vi "Read Synch.vi"(8 "error in (no error)":errorcluster, 11 "AnalogInput in":refnum<class "AnalogInput.lvclass">) -> (0 "error out":errorcluster, 2 "Timing":T1={"Source"="", "Sample Rate (10k)"=10000.0, "sample mode"=10178, "samples per channel"=1000} {"sample mode" items=["Finite Samples"=10178, "Continuous Samples"=10123, "Hardware Timed Single Point"=12522]}, 3 "AnalogInput out":refnum<class "AnalogInput.lvclass">)   [LabVIEW 2019, in "AnalogInput.lvlib" / "AnalogInput.lvclass"]
uses:
  Library/AnalogInput.lvclass
  Custom Controls/Synch Settings.ctl
  Library/AnalogInput.lvclass/AnalogInput.ctl
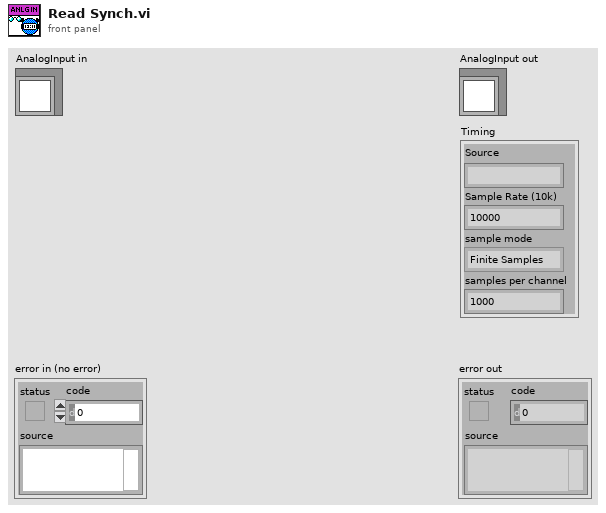
[diagram p1: front panel]
types:
  T1 = typedef "AnalogInput.lvlib/AnalogInput.lvclass/Synch Settings.ctl" = cluster{"Source":string, "Sample Rate (10k)":dbl, "sample mode":i32, "samples per channel":i32}
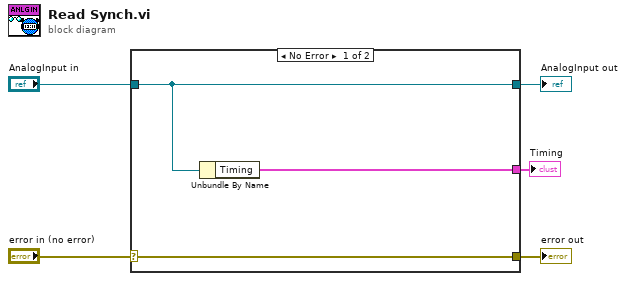
[diagram p0: block diagram]
diagram:
  n1 = case shown="No Error" "error in (no error)" {
    selector: "error in (no error)" -> [w8 w9]
    tunnel: [w8 w9] -> w4
    tunnel: [w7 w10] -> w2
    tunnel: "AnalogInput in" -> [w7 w10]
    tunnel: [w6 _] -> w1
    frame No Error {
      n2 = Unbundle By Name(w7) -> ("Timing"=w6:T1)
    }
    frame Error {
    }
  }
  "error out" <- w4
  "AnalogInput out" <- w2
  "Timing" <- w1
